vi "Read Path.vi"(10 "Error In":errorcluster, 11 "Path .NET Ref":refnum<k24>) -> (2 "Error Out":errorcluster, 3 "Path Properties":T1)   [LabVIEW 2015, in "VeriStand XML Parser.lvlib"]
uses:
  VeriStand XML Parser.lvlib
  NationalInstruments.VeriStand.XMLReader
  XML Controls/Path Cluster.ctl
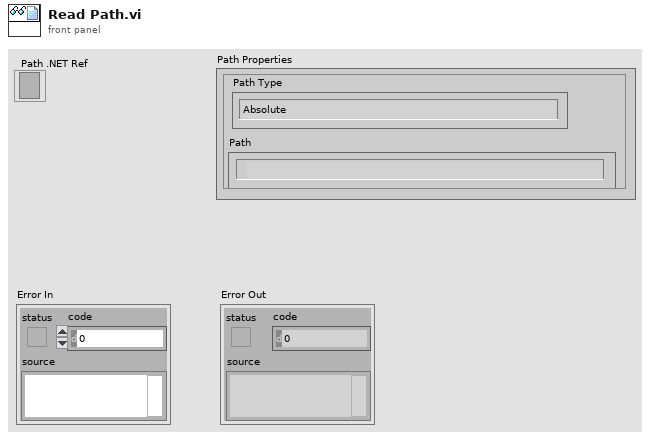
[diagram p1: front panel]
types:
  T1 = typedef "VeriStand XML Parser.lvlib/Path Cluster.ctl" = cluster{"Path":path, "Path Type":enum16{"Absolute", "To Base", "To Common Doc Dir", "To Application Data Dir"}}
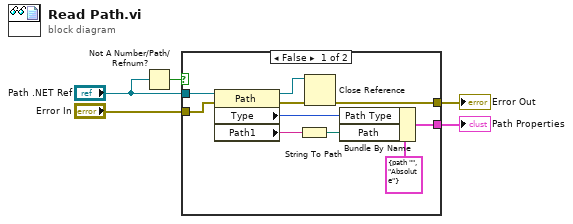
[diagram p0: block diagram]
diagram:
  n1 = Not A Number/Path/Refnum?(number/path/refnum="Path .NET Ref") -> (NaN/Path/Refnum?=w3:bool)
  n2 = case shown="False" w3 {
    tunnel: [w13 w16] -> w5
    tunnel: "Error In" -> [w12 w16]
    tunnel: "Path .NET Ref" -> [w11 _]
    tunnel: [w7 _] -> w1
    frame False {
      n3 = property class="Path"(reference=w11, error in=w12) -> (reference out=w15:refnum<k24>, error out=w14:errorcluster, "Type"=w6:i32, "Path1"=w8:string)
      n4 = String To Path(string=w8) -> (path=w9:path)
      n5 = Close Reference(reference=w15, error in (no error)=w14) -> (error out=w13:errorcluster)
      n6 = Bundle By Name(cluster=T1 {"Path"=path "", "Path Type"=enum."Absolute"} ("Path"), "Path Type"=w6, "Path"=w9) -> (w7:T1)
    }
    frame True {
    }
  }
  "Error Out" <- w5
  "Path Properties" <- w1
